vi "Escape.vi"(7 "Action":enum8{"Escape", "Unescape"}(ring), 11 "String in":string) -> (2 "Has Escape Chars?":bool, 3 "String out":string)   [LabVIEW 2018]
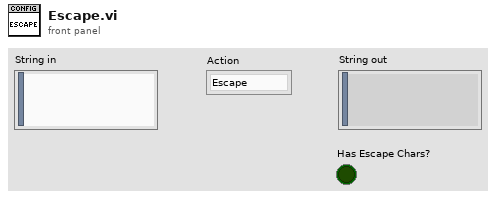
[diagram p1: front panel]
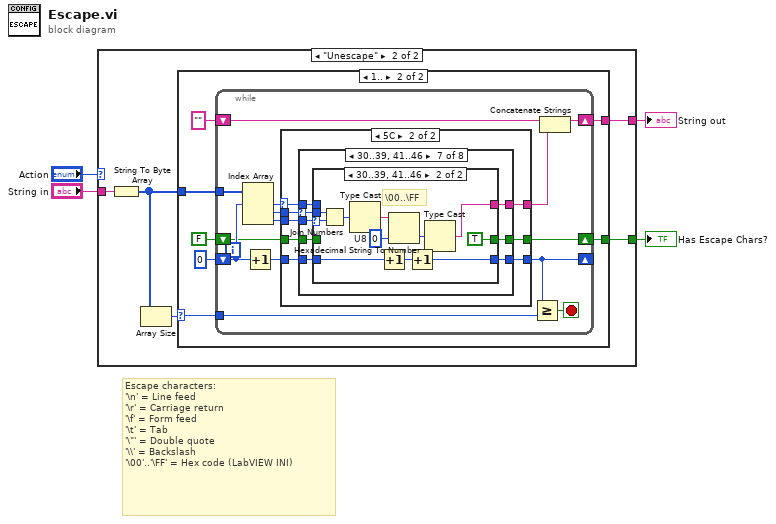
[diagram p0: block diagram]
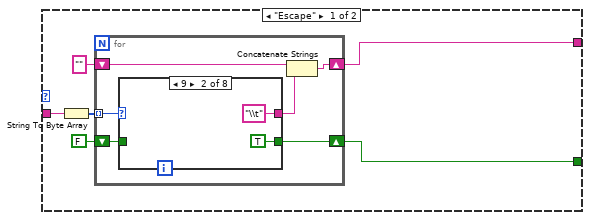
[diagram p2: hidden frame]
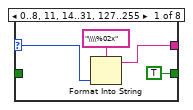
[diagram p3: hidden frame]
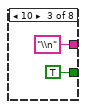
[diagram p4: hidden frame]
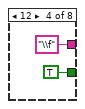
[diagram p5: hidden frame]
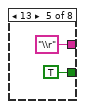
[diagram p6: hidden frame]
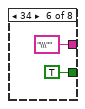
[diagram p7: hidden frame]
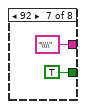
[diagram p8: hidden frame]
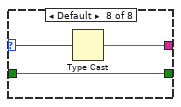
[diagram p9: hidden frame]
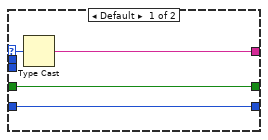
[diagram p11: hidden frame]
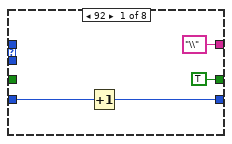
[diagram p12: hidden frame]
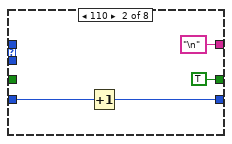
[diagram p13: hidden frame]
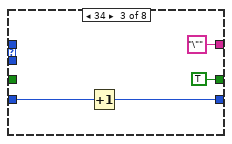
[diagram p14: hidden frame]
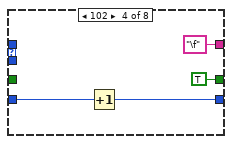
[diagram p15: hidden frame]
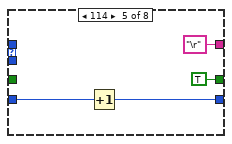
[diagram p16: hidden frame]
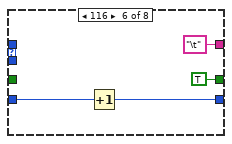
[diagram p17: hidden frame]
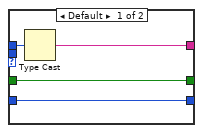
[diagram p18: hidden frame]
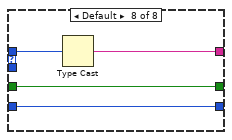
[diagram p19: hidden frame]
diagram:
  # "Escape characters:\n'\\n' = Line feed\n'\\r' = Carriage return\n'\\f' = Form feed\n'\\t' = Tab\n'\\\"' = Double quote\n'\\\\' = Backslash\n'\\00'..'\\FF' = Hex code (LabVIEW INI)"
  n1 = case shown="\"Unescape\"" "Action" {
    tunnel: [w5 w38] -> w4
    tunnel: [w6 w37] -> w3
    tunnel: "String in" -> [w7 w36]
    frame "Escape" {
      n2 = String To Byte Array(string=w7) -> (unsigned byte array=w10:u8[])
      n3 = for {
        tunnel: w10 -> [w16] mode=indexing
        shift-right: [w14] -> w6
        shift-left: "" -> [w15]
        shift-right: [w12] -> w5
        shift-left: FALSE -> [w11]
        n4 = case shown="9" w16 {
          selector: w16 -> [w19 _ _ _ _ _ _ w35]
          tunnel: [w17 "\\t" "\\n" "\\f" "\\r" "\\\"" "\\\\" w34] -> w13
          tunnel: [TRUE TRUE TRUE TRUE TRUE TRUE TRUE w33] -> w12
          tunnel: w11 -> [_ _ _ _ _ _ _ w33]
          frame 0..8, 11, 14..31, 127..255 {
            n5 = Format Into String(format string="\\\\%02x", w19) -> (resulting string=w17:string)  [unwired: 2 in, 1 out]
          }
          frame 9 {
          }
          frame 10 {
          }
          frame 12 {
          }
          frame 13 {
          }
          frame 34 {
          }
          frame 92 {
          }
          frame Default {
            n6 = Type Cast(x=w35) -> (*(type *) &x=w34:string)  [unwired: 1 in]
          }
        }
        n7 = Concatenate Strings(w15, w13) -> (w14:string)
      }
    }
    frame "Unescape" {
      n8 = String To Byte Array(string=w36) -> (unsigned byte array=w39:u8[])
      n9 = Array Size(array=w39) -> (size(s)=w40:i32)
      n10 = case shown="1.." w40 {
        selector: w40 -> [_ w43]
        tunnel: w39 -> [_ w46]
        tunnel: [_ w44] -> w37
        tunnel: [_ w42] -> w38
        frame ..0 {
        }
        frame 1.. {
          n11 = while {
            tunnel: w46 -> [w61]
            shift-right: [w55] -> w44
            shift-left: "" -> [w56]
            shift-right: [w52] -> _
            shift-left: 0 ("index") -> [w60]
            tunnel: w43 -> [w50]
            shift-right: [w49] -> w42
            shift-left: FALSE -> [w48]
            stop <- w51 stop-if-true
            n12 = Index Array(array=w61, index #1=w60) -> (element #1=w59:u8, element #2=w58:u8, element #3=w57:u8)  [unwired: 2 in]
            n13 = Increment(x=w60) -> (x+1=w53:i32)
            n14 = case shown="5C" w59 {
              selector: w59 -> [w65 w72]
              tunnel: w58 -> [_ w73]
              tunnel: w57 -> [_ w70]
              tunnel: [w64 w71] -> w54
              tunnel: [w63 w69] -> w52
              tunnel: w53 -> [w63 w68]
              tunnel: [w62 w67] -> w49
              tunnel: w48 -> [w62 w66]
              frame Default {
                n15 = Type Cast(x=w65) -> (*(type *) &x=w64:string)  [unwired: 1 in]
              }
              frame 92 {
                n16 = case shown="30..39, 41..46" w73 {
                  selector: w73 -> [_ _ _ _ _ _ w105 _]
                  tunnel: w72 -> [_ _ _ _ _ _ w103 w124]
                  tunnel: ["\\" "\n" "\"" "\f" "\r" "\t" w102 w123] -> w71
                  tunnel: w70 -> [_ _ _ _ _ _ w104 _]
                  tunnel: [w75 w79 w83 w87 w91 w95 w101 w122] -> w69
                  tunnel: w68 -> [w76 w80 w84 w88 w92 w96 w100 w122]
                  tunnel: [TRUE TRUE TRUE TRUE TRUE TRUE w99 w121] -> w67
                  tunnel: w66 -> [_ _ _ _ _ _ w98 w121]
                  frame 92 {
                    n17 = Increment(x=w76) -> (x+1=w75:i32)
                  }
                  frame 110 {
                    n18 = Increment(x=w80) -> (x+1=w79:i32)
                  }
                  frame 34 {
                    n19 = Increment(x=w84) -> (x+1=w83:i32)
                  }
                  frame 102 {
                    n20 = Increment(x=w88) -> (x+1=w87:i32)
                  }
                  frame 114 {
                    n21 = Increment(x=w92) -> (x+1=w91:i32)
                  }
                  frame 116 {
                    n22 = Increment(x=w96) -> (x+1=w95:i32)
                  }
                  frame 48..57, 65..70 {
                    n23 = case shown="30..39, 41..46" w104 {
                      selector: w104 -> [_ w119]
                      tunnel: w105 -> [_ w120]
                      tunnel: w103 -> [w109 _]
                      tunnel: [w108 w114] -> w102
                      tunnel: [w107 w111] -> w101
                      tunnel: w100 -> [w107 w113]
                      tunnel: [w106 TRUE] -> w99
                      tunnel: w98 -> [w106 _]
                      frame Default {
                        n24 = Type Cast(x=w109) -> (*(type *) &x=w108:string)  [unwired: 1 in]
                      }
                      frame 48..57, 65..70 {
                        w116 = u8 0  # U8
                        # "\\00..\\FF"
                        n25 = Join Numbers(hi=w120, lo=w119) -> ((hi.lo)=w118:u16)
                        n26 = Type Cast(x=w118) -> (*(type *) &x=w117:string)  [unwired: 1 in]
                        n27 = Increment(x=w113) -> (x+1=w112:i32)
                        n28 = Hexadecimal String To Number(string=w117, default (0uL)=w116) -> (number=w115:u8)  [unwired: 1 in, 1 out]
                        n29 = Increment(x=w112) -> (x+1=w111:i32)
                        n30 = Type Cast(x=w115) -> (*(type *) &x=w114:string)  [unwired: 1 in]
                      }
                    }
                  }
                  frame Default {
                    n31 = Type Cast(x=w124) -> (*(type *) &x=w123:string)  [unwired: 1 in]
                  }
                }
              }
            }
            n32 = Greater Or Equal?(x=w52, y=w50) -> (x >= y?=w51:bool)
            n33 = Concatenate Strings(w56, w54) -> (w55:string)
          }
        }
      }
    }
  }
  "String out" <- w3
  "Has Escape Chars?" <- w4
